vi "Store Unit of Work.vi"(7 "Unit Of Work":refnum<class "Unit Of Work Session.lvclass">, 11 "Entity Manager in":refnum<class "Entity Manager.lvclass">) -> (3 "Entity Manager out":refnum<class "Entity Manager.lvclass">)   [LabVIEW 2020, in "Conditu2.lvlib" / "Entity Manager.lvclass"]
uses:
  Entity Manager.lvclass
  Unit Of Work Session/Unit Of Work Session.lvclass
  Entity Manager.lvclass/Entity Manager.ctl
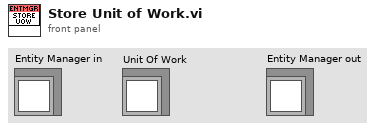
[diagram p1: front panel]
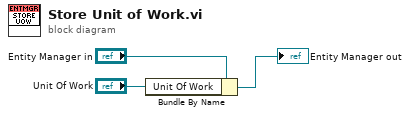
[diagram p0: block diagram]
diagram:
  n1 = Bundle By Name(cluster="Entity Manager in", "Unit Of Work"="Unit Of Work") -> (→"Entity Manager out":refnum<class "Entity Manager.lvclass">)
